vi "Fits_control_stage.vi"() -> ()   [LabVIEW 2018]
uses:
  <vilib>/express/express arith-compare/Formula/XNode/ExpressFormulaBlockNode.xnode
  DLL/XMT_DLL_SER.dll
  wlmData.dll
panel:
  out "RData 3":sgl
  out "RData 2":sgl
  in  "电机安装偏差角度":dbl
  in  "ReFlag 5":u8
  out "error out":errorcluster
  in  "波长计\nChannel":i32
  out "wavelength / nm":dbl format="%#_18f"
  out "获取到的信号光波长":dbl
  out "lam_signal(nm)":dbl
  in  "停止":bool
  in  "Ch":u8
  in  "Address":u8=1
  out "lam_idler(o) (nm)":dbl
  out "lam_shg(e) (nm)":dbl
  in  "COM":u64=3
  out "int":i8
  out "返回类型":u8
  out "错误输出":errorcluster
  # "电机"
  # "信号光波长有效值"
  # "开环O:79"
  # "闭环C:67"
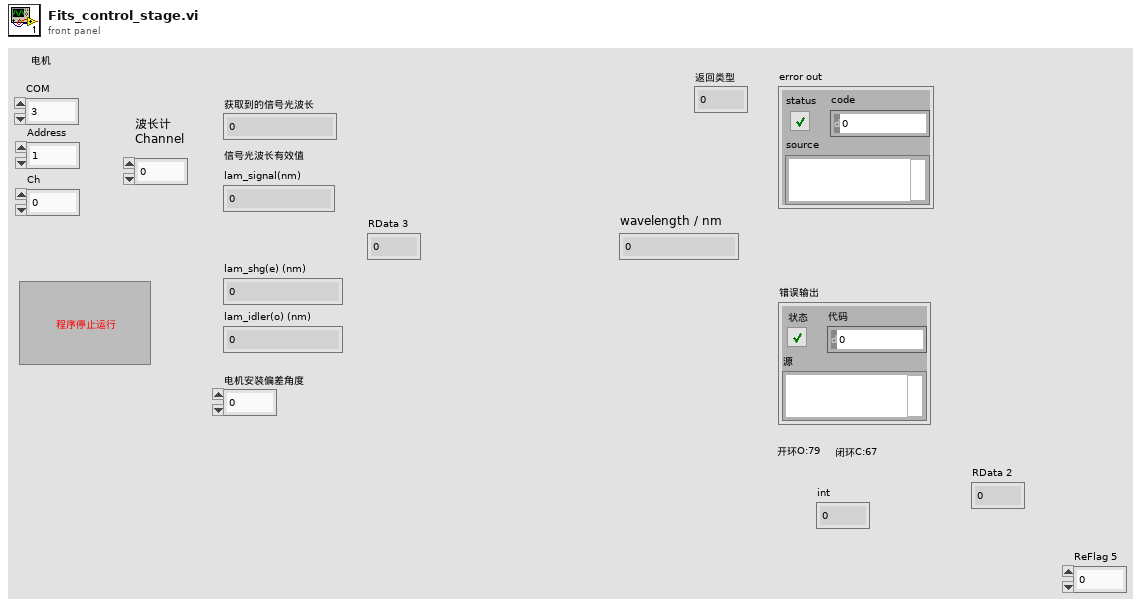
[diagram p1: front panel]
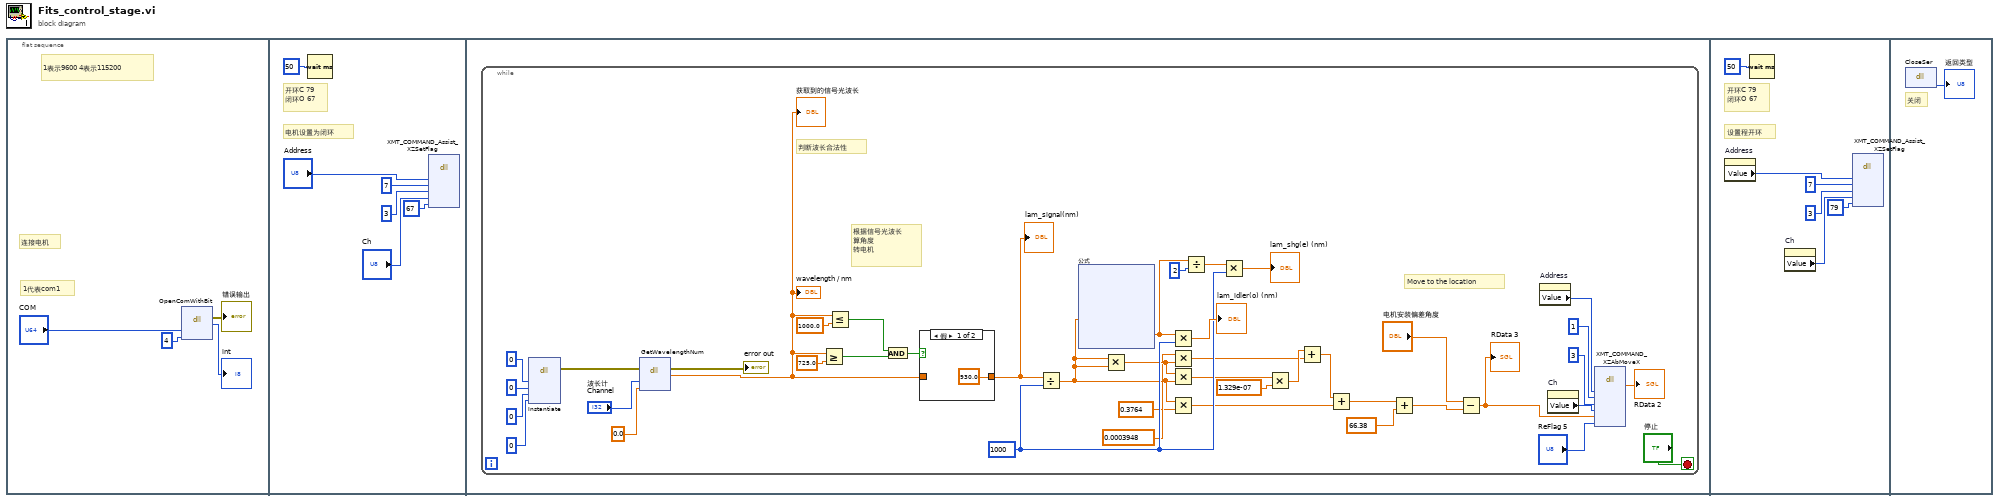
[diagram p0: block diagram]
diagram:
  n1 = flat-sequence {
    frame #0 {
      # "连接电机"
      # "1表示9600 4表示115200"
      # "1代表com1"
      n2 = dll-call lib="C:/Users/cy3486/OneDrive/Desktop/OPO_control_scripts/SHG_motor_control/DLL/XMT_DLL_SER.dll" fn="OpenComWithBit"("m_com"="COM", "BaudRate"=u8 4) -> (error out=→"错误输出":errorcluster, "int"=→"int":i8)  [unwired: 5 in, 1 out]
    }
    frame #1 {
      # "电机设置为闭环"
      # "开环C 79\n闭环O 67"
      n3 = Wait (ms)(milliseconds to wait=u32 50 ("等待时间（毫秒）")) -> ()  [unwired: 1 out]
      n4 = dll-call lib="C:/Users/cy3486/OneDrive/Desktop/OPO_control_scripts/SHG_motor_control/DLL/XMT_DLL_SER.dll" fn="XMT_COMMAND_Assist_XZSetFlag"("Address"="Address", "Command_B3"=u16 7, "Command_B4"=u16 3 ("Command_B3"), "Ch"="Ch", "SetFalg"=67) -> ()  [unwired: 9 in, 2 out]
    }
    frame #2 {
      n5 = while {
        stop <- "停止" stop-if-true
        w48 = 1000
        # "Move to the location"
        # "判断波长合法性"
        # "根据信号光波长\n算角度\n转电机"
        n6 = dll-call lib="wlmData.dll" fn="Instantiate"("arg1"=u32 0, "arg2"=0, "arg3"=u32 0, "arg4"=u32 0) -> (error out=w34:errorcluster)  [unwired: 8 in, 1 out]
        n7 = dll-call lib="wlmData.dll" fn="GetWavelengthNum"(error in=w34, "arg1"="波长计\nChannel", "arg2"=0.0) -> (error out=→"error out":errorcluster, "return type"=w35:dbl)  [unwired: 4 in, 1 out]
        "获取到的信号光波长" <- w35
        "wavelength / nm" <- w35
        n8 = Greater Or Equal?(x=w35, y=725.0) -> (x >= y?=w44:bool)
        n9 = Less Or Equal?(x=w35, y=1000.0) -> (x <= y?=w45:bool)
        n10 = And(x=w45, y=w44) -> (x .and. y?=w46:bool)
        n11 = case shown="假" w46 {
          tunnel: [930.0 w55] -> w41
          tunnel: w35 -> [_ w55]
          frame False {
          }
          frame True {
          }
        }
        "lam_signal(nm)" <- w41
        n12 = Divide(x=w41, y=w48) -> (x/y=w16:dbl)
        n13 = xnode "公式"("lam"=w16) -> ("结果"=w49:dbl)  [unwired: 1 in, 1 out]
        n14 = Multiply(x=w16, y=w16) -> (x*y=w21:dbl)
        n15 = Multiply(x=w49, y=w48) -> (x*y=→"lam_idler(o) (nm)":dbl)
        n16 = Multiply(x=0.0003948, y=w21) -> (x*y=w19:dbl)
        n17 = Multiply(x=w21, y=w16) -> (x*y=w24:dbl)
        n18 = Multiply(x=w16, y=0.3764) -> (x*y=w14:dbl)
        n19 = Divide(x=w49, y=2) -> (x/y=w52:dbl)
        n20 = Multiply(x=w52, y=w48) -> (x*y=→"lam_shg(e) (nm)":dbl)
        n21 = Multiply(x=w24, y=1.329e-07) -> (x*y=w22:dbl)
        n22 = Add(x=w22, y=w19) -> (x+y=w18:dbl)
        n23 = Add(x=w18, y=w14) -> (x+y=w17:dbl)
        n24 = Add(x=w17, y=66.38) -> (x+y=w12:dbl)
        n25 = Subtract(x="电机安装偏差角度", y=w12) -> (x-y=w11:dbl)
        "RData 3" <- w11
        n26 = property on="Address" class="DigNum (严格)"() -> ("Value"=w30:u8)  [unwired: 2 in, 2 out]
        n27 = property on="Ch" class="DigNum (严格)"() -> ("Value"=w29:u8)  [unwired: 2 in, 2 out]
        n28 = dll-call lib="C:/Users/cy3486/OneDrive/Desktop/OPO_control_scripts/SHG_motor_control/DLL/XMT_DLL_SER.dll" fn="XMT_COMMAND_XZAbMoveX"("Address"=w30, "Command_B3"=u16 1, "Command_B4"=u16 3 ("Command_B3"), "Ch"=w29, "MoveX_f"=w11, "ReFlag"="ReFlag 5") -> ("RData"=→"RData 2":sgl)  [unwired: 9 in, 2 out]
      }
    }
    frame #3 {
      # "设置程开环"
      # "开环C 79\n闭环O 67"
      n29 = property on="Address" class="DigNum (严格)"() -> ("Value"=w65:u8)  [unwired: 2 in, 2 out]
      n30 = Wait (ms)(milliseconds to wait=u32 50 ("等待时间（毫秒）")) -> ()  [unwired: 1 out]
      n31 = property on="Ch" class="DigNum (严格)"() -> ("Value"=w64:u8)  [unwired: 2 in, 2 out]
      n32 = dll-call lib="C:/Users/cy3486/OneDrive/Desktop/OPO_control_scripts/SHG_motor_control/DLL/XMT_DLL_SER.dll" fn="XMT_COMMAND_Assist_XZSetFlag"("Address"=w65, "Command_B3"=u16 7, "Command_B4"=u16 3 ("Command_B3"), "Ch"=w64, "SetFalg"=79) -> ()  [unwired: 9 in, 2 out]
    }
    frame #4 {
      # "关闭"
      n33 = dll-call lib="C:/Users/cy3486/OneDrive/Desktop/OPO_control_scripts/SHG_motor_control/DLL/XMT_DLL_SER.dll" fn="CloseSer"() -> ("返回类型"=→"返回类型":u8)  [unwired: 3 in, 2 out]
    }
  }
